vi "LVClass_Image Image Load.vi"(0 "Image in":refnum<class "Image.lvclass">, 5 "path":path, 11 "error in (no error)":errorcluster) -> (4 "Image out":refnum<class "Image.lvclass">, 15 "error out":errorcluster)   [LabVIEW 2020, in "Image.lvclass"]
doc: "Load Image from file.\n\n--------------------------------------------------------------------------------\n\n<B>ImageIn </B> : Image object.\n<B>ImageOut </B> : Image object.\n<B>image_file_path </B> : Absolute path to image file.\n<B>ErrorIn </B> : Error\n<B>ErrorOut </B> : Error\n\n--------------------------------------------------------------------------------"
uses:
  Image.lvclass
  Image.lvclass/Image.ctl
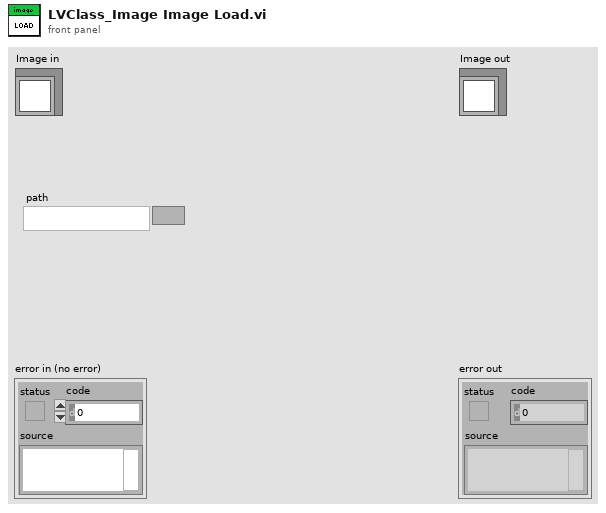
[diagram p1: front panel]
types:
  T1 = typedef "ClassID.ctl" = i64
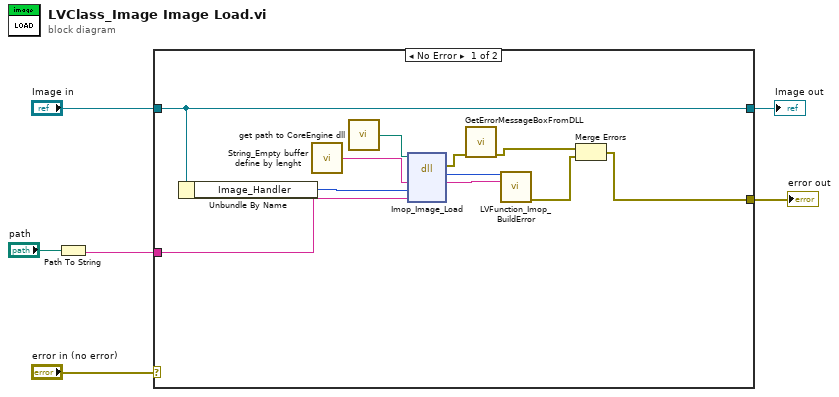
[diagram p0: block diagram]
diagram:
  n1 = Path To String(path="path") -> (string=w1:string)
  n2 = case shown="No Error" "error in (no error)" {
    selector: "error in (no error)" -> [_ w19]
    tunnel: [w7 w19] -> w5
    tunnel: [w13 w18] -> w3
    tunnel: "Image in" -> [w13 w18]
    tunnel: w1 -> [w10 _]
    frame No Error {
      n3 = Unbundle By Name(w13) -> ("Image_Handler"=w14:T1)
      n4 = call "String_Empty buffer define by lenght.vi"() -> ("Empty buffer"=w17:string)  [unwired: 1 in]
      n5 = call "get path to CoreEngine dll.vi"() -> ("path to wavekit library"=w12:path)  [unwired: 14 in, 1 out]
      n6 = dll-call lib="D:/2_trunk/Soft_haso/ImOpCoreEngine4_LV2011/DLLs/ImopEngine4_vc100.dll" fn="Imop_Image_Load"(path in=w12, "message"=w17, "Image compat"=w14, "path"=w10) -> (error out=w11:errorcluster, "return type"=w16:i32, "message"=w15:string)  [unwired: 4 in, 1 out]
      n7 = call "GetErrorMessageBoxFromDLL.vi"("error IN"=w11) -> ("error OUT"=w9:errorcluster)  [unwired: 10 in]
      n8 = call "LVFunction_Imop_BuildError.vi"("code"=w16, "String to Prepend to source (\"\")"=w15) -> ("error out"=w8:errorcluster)  [unwired: 13 in]
      n9 = Merge Errors(w9, w8) -> (w7:errorcluster)
    }
    frame Error {
    }
  }
  "error out" <- w5
  "Image out" <- w3
